vi "TDMS Copy Properties.vi"(5 "channel name":string, 7 "group name":string, 8 "error in":errorcluster, 10 "tdms dest in":refnum<k34>, 11 "tdms source in":refnum<k34>) -> (0 "error out":errorcluster, 2 "tdms dest out":refnum<k34>, 3 "tdms source out":refnum<k34>)   [LabVIEW 2011]
doc: "Copies all the file, group or channel properties from the source file to the est file."
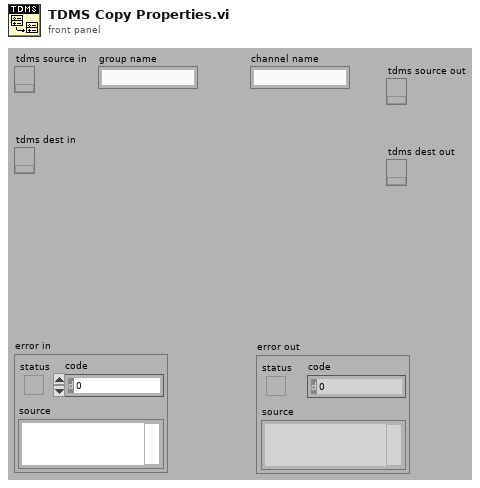
[diagram p1: front panel]
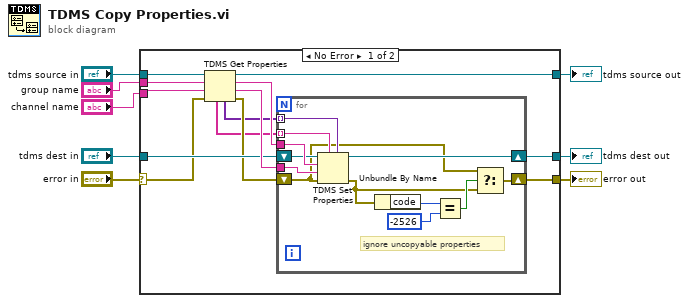
[diagram p0: block diagram]
diagram:
  n1 = case shown="No Error" "error in" {
    selector: "error in" -> [w14 w35]
    tunnel: [w13 w35] -> w8
    tunnel: "tdms source in" -> [w21 w36]
    tunnel: [w20 w36] -> w6
    tunnel: "group name" -> [w19 _]
    tunnel: "tdms dest in" -> [w16 w34]
    tunnel: "channel name" -> [w15 _]
    tunnel: [w9 w34] -> w1
    frame No Error {
      n2 = TDMS Get Properties(8:w14, 9:w15, 10:w19, 11:w21) -> (0:w12:errorcluster, 1:w17:string, 2:w18:string, 3:w20:refnum<k34>, 4:w11:variant[], 6:w10:string[])  [unwired: 2 out]
      n3 = for {
        tunnel: w18 -> [w33]
        tunnel: w17 -> [w32]
        tunnel: w11 -> [w30] mode=indexing
        tunnel: w10 -> [w29] mode=indexing
        shift-right: [w24] -> w13
        shift-left: w12 -> [w23]
        shift-right: [w28] -> w9
        shift-left: w16 -> [w31]
        # "ignore uncopyable properties"
        n4 = TDMS Set Properties(5:w30, 7:w29, 8:w23, 9:w32, 10:w33, 11:w31) -> (0:w22:errorcluster, 3:w28:refnum<k34>)  [unwired: 2 out]
        n5 = Unbundle By Name(w22) -> ("code"=w27:i32)
        n6 = Equal?(x=w27, y=-2526) -> (x = y?=w25:bool)
        n7 = Select(t=w23, s=w25, f=w22) -> (s? t:f=w24:errorcluster)
      }
    }
    frame Error {
    }
  }
  "error out" <- w8
  "tdms source out" <- w6
  "tdms dest out" <- w1
